vi "Configure BERT Route Source.vi"(6 "Gate Source (1: None)":i32(ring)=1 items=["BB Trigger2", "None"], 7 "Data Source (1: None)":i32(ring)=1 items=["Event1", "None"], 8 "error in (no error)":errorcluster, 9 "Clock Source (1: None)":i32(ring)=1 items=["BB Trigger1", "None"], 10 "BERT Route Source (0: Gate)":i32(ring) items=["Gate", "Clock", "Data"], 11 "VISA resource name":refnum<visa-resource-name>) -> (0 "error out":errorcluster, 3 "VISA resource name out":refnum<visa-resource-name>)   [LabVIEW 2018, in "Agilent PSG MXG Series.lvlib"]
doc: "Configures route source of bit error rate.\n\n<b>Note:</b>\nIt is applicable for N5172B/82B with <b>Option UN7</b> only."
uses:
  Agilent PSG MXG Series.lvlib
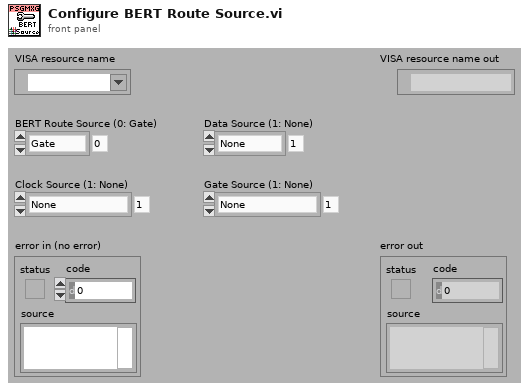
[diagram p1: front panel]
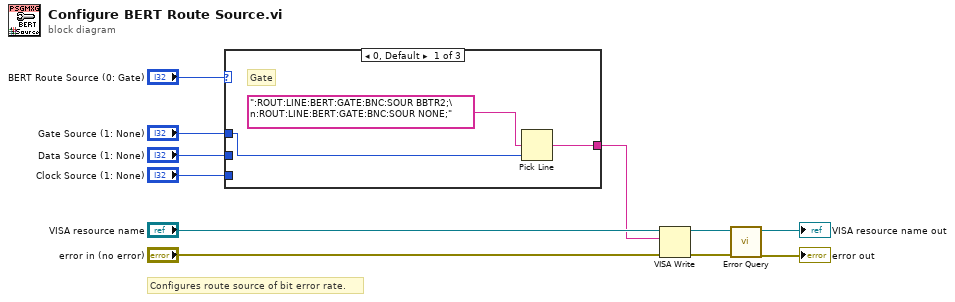
[diagram p0: block diagram]
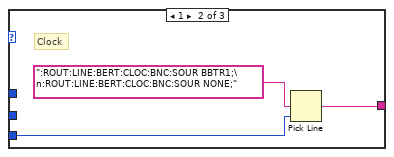
[diagram p2: hidden frame]
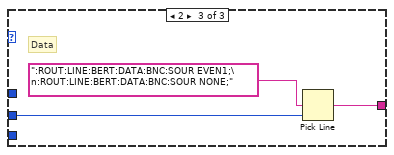
[diagram p3: hidden frame]
diagram:
  # "Configures route source of bit error rate."
  n1 = case shown="0, Default" "BERT Route Source (0: Gate)" {
    tunnel: "Data Source (1: None)" -> [_ _ w19]
    tunnel: [w13 w16 w18] -> w4
    tunnel: "Clock Source (1: None)" -> [_ w15 _]
    tunnel: "Gate Source (1: None)" -> [w12 _ _]
    frame 0, Default {
      # "Gate"
      n2 = Pick Line(multi-line string=":ROUT:LINE:BERT:GATE:BNC:SOUR BBTR2;\n:ROUT:LINE:BERT:GATE:BNC:SOUR NONE;", line index=w12) -> (output string=w13:string)  [unwired: 1 in]
    }
    frame 1 {
      # "Clock"
      n3 = Pick Line(multi-line string=":ROUT:LINE:BERT:CLOC:BNC:SOUR BBTR1;\n:ROUT:LINE:BERT:CLOC:BNC:SOUR NONE;", line index=w15) -> (output string=w16:string)  [unwired: 1 in]
    }
    frame 2 {
      # "Data"
      n4 = Pick Line(multi-line string=":ROUT:LINE:BERT:DATA:BNC:SOUR EVEN1;\n:ROUT:LINE:BERT:DATA:BNC:SOUR NONE;", line index=w19) -> (output string=w18:string)  [unwired: 1 in]
    }
  }
  n5 = VISA Write(VISA resource name="VISA resource name", write buffer=w4, error in (no error)="error in (no error)") -> (VISA resource name out=w9:refnum<visa-resource-name>, error out=w8:errorcluster)  [unwired: 1 out]
  n6 = call "Error Query.vi"("error in (no error)"=w8, "VISA resource name"=w9) -> ("error out"=→"error out":errorcluster, "VISA resource name out"=→"VISA resource name out":refnum<visa-resource-name>)  [unwired: 6 in, 2 out]
